vi "Build Report String.vi"(8 "error in (no error)":errorcluster, 10 "Report Data":T1, 11 "Keyboard Macro in":refnum<class "Keyboard Macro.lvclass">) -> (0 "error out":errorcluster, 2 "Report String":string, 3 "Keyboard Macro out":refnum<class "Keyboard Macro.lvclass">)   [LabVIEW 2020, in "MacroAssert.lvlib" / "Keyboard Macro.lvclass"]
doc: "Builds a string using <B>Step</B> and <B>Report Data</B> to be included in a report."
uses:
  Keyboard Macro.lvclass
  Keyboard Macro.lvclass/Keyboard Macro.ctl
  CTLs/Report Data.ctl
  MacroAssert.lvlib
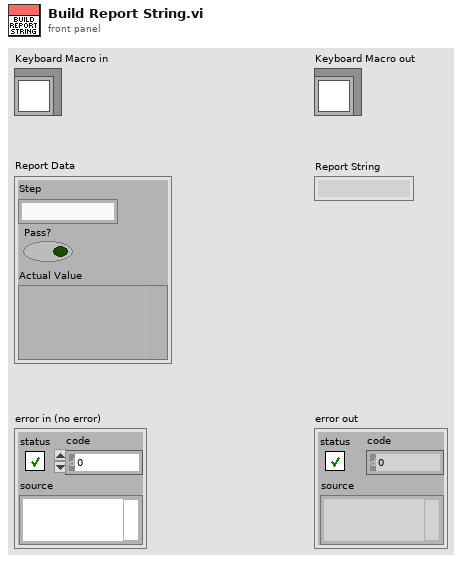
[diagram p1: front panel]
types:
  T1 = typedef "MacroAssert.lvlib/Report Data.ctl" = cluster{"Step":string, "Pass?":bool, "Actual Value":variant}
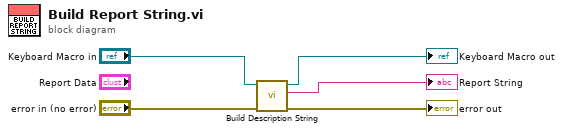
[diagram p0: block diagram]
diagram:
  n1 = call-dynamic "Build Description String.vi"("error in (no error)"="error in (no error)", "Keyboard Macro in"="Keyboard Macro in") -> ("error out"=→"error out":errorcluster, "Description"=→"Report String":string, "Keyboard Macro out"=→"Keyboard Macro out":refnum<class "Keyboard Macro.lvclass">)  [unwired: 7 in]
